vi "Request Data JSON.vi"(8 "error in (no error)":errorcluster, 11 "GetInputList in":refnum<class "GetInputList.lvclass">) -> (0 "error out":errorcluster, 2 "Request Data JSON":string, 3 "GetInputList out":refnum<class "GetInputList.lvclass">)   [LabVIEW 2020, in "obs-websocket.lvlib" / "GetInputList.lvclass"]
uses:
  GetInputList.lvclass
  GetInputList.lvclass/GetInputList.ctl
  a25a6396-fb9c-445d-bee9-698f8707f2bc.vi
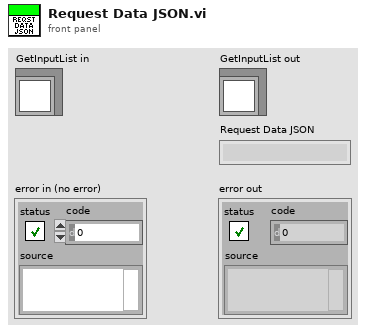
[diagram p1: front panel]
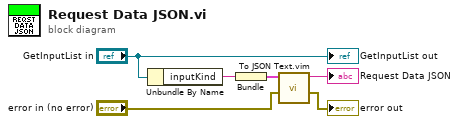
[diagram p0: block diagram]
diagram:
  n1 = Unbundle By Name("GetInputList in") -> ("inputKind"=w5:string)
  n2 = Bundle("inputKind"=w5) -> (w4:cluster{"inputKind":string})  [unwired: 1 in]
  n3 = call "To JSON Text.vim"("error in (no error)"="error in (no error)", "Anything"=w4) -> ("error out"=→"error out":errorcluster, "<JSON>"=→"Request Data JSON":string)  [unwired: 8 in]
  "GetInputList out" <- "GetInputList in"
